vi "KE622x -- Get List Sweep Steps.vi"(0 "Resource In":refnum<visa-resource-name>, 1 "Check For SCPI Errors? (T)":bool=TRUE, 11 "error in (no error)":errorcluster) -> (4 "Resource Out (dupl)":refnum<visa-resource-name>, 8 "List Sweep Steps":T1 {"Current Level (A)" min=-0.105 max=0.105 format="%.4p"; "Source Delay (s)" min=0.001 max=1000.0 step=0.001 format="%.3f"; "Voltage Limit (V)" min=0.1 max=105.0 step=0.01 format="%.2p"}, 10 "Num List Steps":u32, 15 "error out":errorcluster)   [LabVIEW 2019, in "Keithley 622x.lvlib"]
doc: "Returns the individual points in the currently defined list current sweep."
uses:
  Keithley 622x.lvlib
  Typedefs/KE622x -- List Sweep Steps.ctl
  Typedefs/KE622x -- List Sweep Step.ctl
  Typedefs/KE622x -- Current Level.ctl
  Typedefs/KE622x -- Source Delay.ctl
  Typedefs/KE622x -- Voltage Limit.ctl
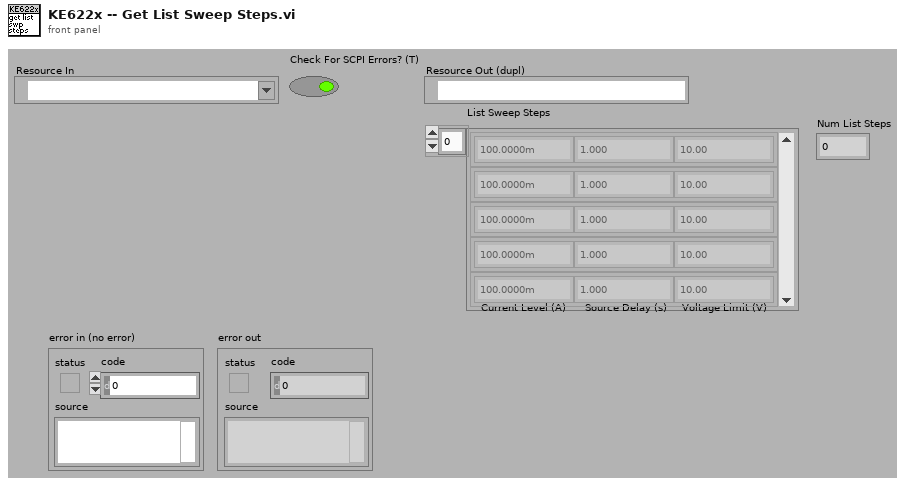
[diagram p1: front panel]
types:
  T1 = typedef "Keithley 622x.lvlib/KE622x -- List Sweep Steps.ctl" = T2[]
  T2 = typedef "Keithley 622x.lvlib/KE622x -- List Sweep Step.ctl" = cluster{"Current Level (A)":T3, "Source Delay (s)":T4, "Voltage Limit (V)":T5}
  T3 = typedef "Keithley 622x.lvlib/KE622x -- Current Level.ctl" = dbl
  T4 = typedef "Keithley 622x.lvlib/KE622x -- Source Delay.ctl" = dbl
  T5 = typedef "Keithley 622x.lvlib/KE622x -- Voltage Limit.ctl" = dbl
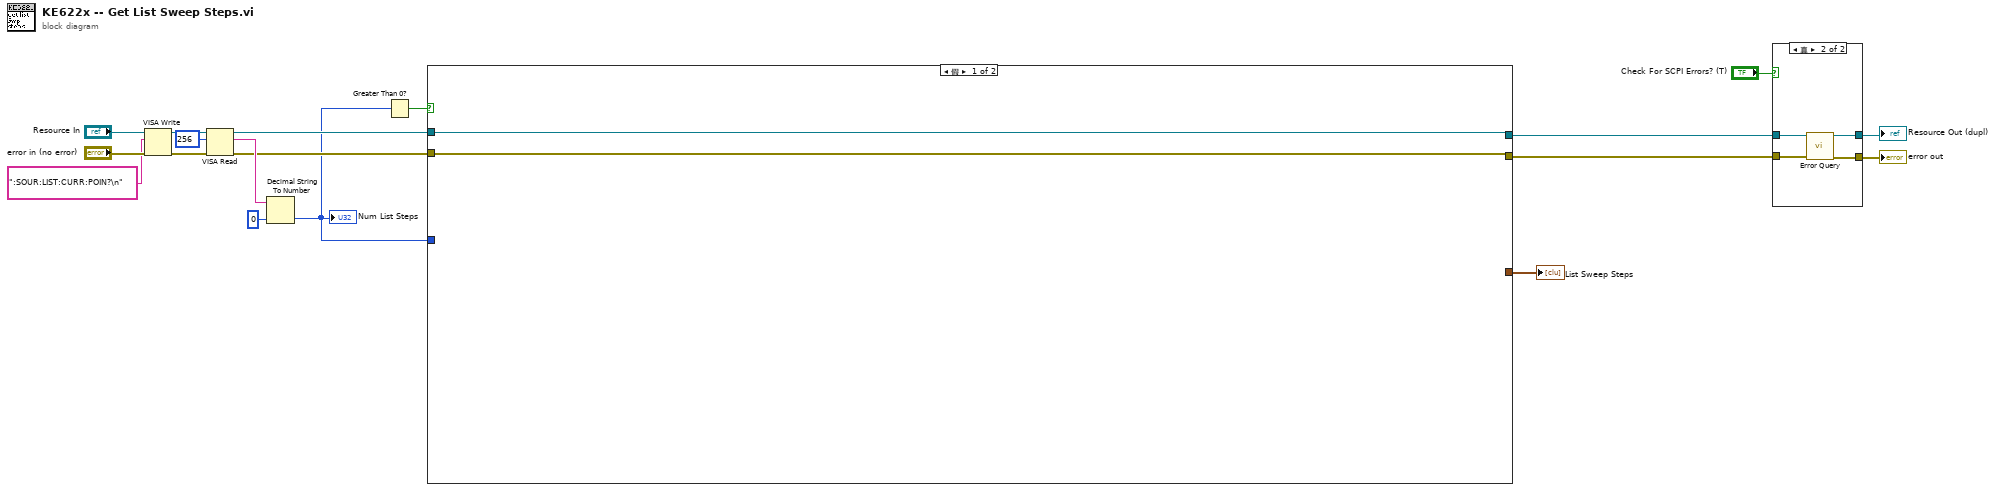
[diagram p0: block diagram]
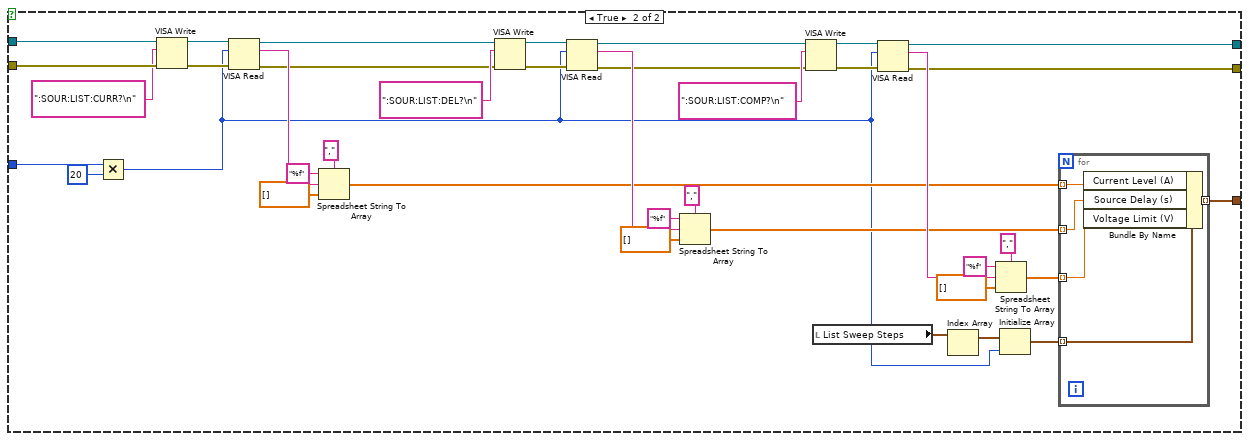
[diagram p2: hidden frame]
diagram:
  n1 = VISA Write(VISA resource name="Resource In", write buffer=":SOUR:LIST:CURR:POIN?\n" ("format string"), error in (no error)="error in (no error)") -> (VISA resource name out=w12:refnum<visa-resource-name>, error out=w11:errorcluster)  [unwired: 1 out]
  n2 = VISA Read(VISA resource name=w12, byte count=u32 256, error in (no error)=w11) -> (VISA resource name out=w7:refnum<visa-resource-name>, read buffer=w9:string, error out=w6:errorcluster)  [unwired: 1 out]
  n3 = Decimal String To Number(string=w9, default (0L)=u32 0 ("default (0 I32)")) -> (number=w3:u32)  [unwired: 1 in, 1 out]
  "Num List Steps" <- w3
  n4 = Greater Than 0?(x=w3) -> (x > 0?=w2:bool)
  n5 = case shown="假" w2 {
    tunnel: w7 -> [w20 w59]
    tunnel: w6 -> [w19 w58]
    tunnel: w3 -> [_ w56]
    tunnel: [w20 w31] -> w5
    tunnel: [w19 w30] -> w4
    tunnel: [_ w21] -> w1
    frame False {
    }
    frame True {
      n6 = Multiply(x=w56, y=u32 20) -> (x*y=w23:u32)
      n7 = VISA Write(VISA resource name=w59, write buffer=":SOUR:LIST:CURR?\n" ("format string"), error in (no error)=w58) -> (VISA resource name out=w54:refnum<visa-resource-name>, error out=w53:errorcluster)  [unwired: 1 out]
      n8 = VISA Read(VISA resource name=w54, byte count=w23, error in (no error)=w53) -> (VISA resource name out=w45:refnum<visa-resource-name>, read buffer=w52:string, error out=w44:errorcluster)  [unwired: 1 out]
      n9 = Spreadsheet String To Array(delimiter (Tab)=",", format string="%f", spreadsheet string=w52, array type (2D Dbl)=dbl[] []) -> (array=w29:dbl[])
      n10 = VISA Write(VISA resource name=w45, write buffer=":SOUR:LIST:DEL?\n" ("format string"), error in (no error)=w44) -> (VISA resource name out=w47:refnum<visa-resource-name>, error out=w46:errorcluster)  [unwired: 1 out]
      n11 = VISA Read(VISA resource name=w47, byte count=w23, error in (no error)=w46) -> (VISA resource name out=w36:refnum<visa-resource-name>, read buffer=w40:string, error out=w35:errorcluster)  [unwired: 1 out]
      n12 = Spreadsheet String To Array(delimiter (Tab)=",", format string="%f", spreadsheet string=w40, array type (2D Dbl)=dbl[] []) -> (array=w28:dbl[])
      n13 = VISA Write(VISA resource name=w36, write buffer=":SOUR:LIST:COMP?\n" ("format string"), error in (no error)=w35) -> (VISA resource name out=w38:refnum<visa-resource-name>, error out=w37:errorcluster)  [unwired: 1 out]
      n14 = local read "List Sweep Steps"() -> (w25:T1)
      n15 = VISA Read(VISA resource name=w38, byte count=w23, error in (no error)=w37) -> (VISA resource name out=w31:refnum<visa-resource-name>, read buffer=w32:string, error out=w30:errorcluster)  [unwired: 1 out]
      n16 = Index Array(array=w25) -> (element=w24:T2)  [unwired: 1 in]
      n17 = Spreadsheet String To Array(delimiter (Tab)=",", format string="%f", spreadsheet string=w32, array type (2D Dbl)=dbl[] []) -> (array=w27:dbl[])
      n18 = Initialize Array(w24, w23) -> (w22:T2[])
      n19 = for {
        tunnel: w29 -> [w63] mode=indexing
        tunnel: w28 -> [w62] mode=indexing
        tunnel: w27 -> [w61] mode=indexing
        tunnel: w22 -> [w64] mode=indexing
        tunnel: [w60] -> w21 mode=indexing
        n20 = Bundle By Name(cluster=w64, "Current Level (A)"=w63, "Source Delay (s)"=w62, "Voltage Limit (V)"=w61) -> (w60:T2)
      }
    }
  }
  "List Sweep Steps" <- w1
  n21 = case shown="真" "Check For SCPI Errors? (T)" {
    tunnel: w5 -> [w66 w70]
    tunnel: [w65 w69] -> w14
    tunnel: [w66 w68] -> w15
    tunnel: w4 -> [w65 w67]
    frame False {
    }
    frame True {
      n22 = call "Error Query.vi"("VISA Resource In"=w70, "error in (no error)"=w67) -> ("VISA Resource Out (dupl)"=w68:refnum<visa-resource-name>, "error out"=w69:errorcluster)  [unwired: 10 in, 2 out]
    }
  }
  "Resource Out (dupl)" <- w15
  "error out" <- w14
